vi "Convert_rpm_V.vi"(10 "Speed Set Point (rpm)":dbl format="%#_13g") -> (2 "?":dbl format="%#_13g")   [LabVIEW 2014]
panel:
  # "Scaling Motor speed [rpm - V]"
  # "Output Voltage"
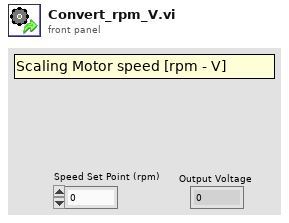
[diagram p1: front panel]
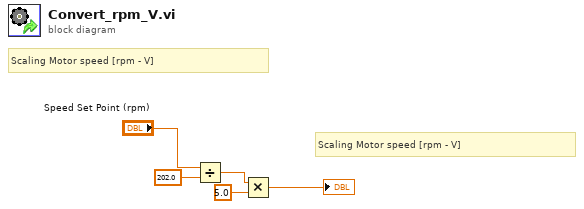
[diagram p0: block diagram]
diagram:
  # "Scaling Motor speed [rpm - V]"
  # "Scaling Motor speed [rpm - V]"
  n1 = Divide(x="Speed Set Point (rpm)", y=202.0 ("Speed Set Point (rpm) 2")) -> (x/y=w4:dbl)
  n2 = Multiply(x=w4, y=5.0 ("Speed Set Point (rpm) 2")) -> (x*y=→"?":dbl)
